vi "Test Section Cluster Tools.vi"() -> ()   [LabVIEW 2015]
uses:
  JSONtext.lvlib
panel:
  out "data":cluster{"3124":i32, "efqwf":string}
  out "error out":errorcluster
  out "<JSON>":string
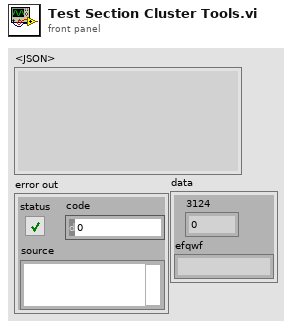
[diagram p1: front panel]
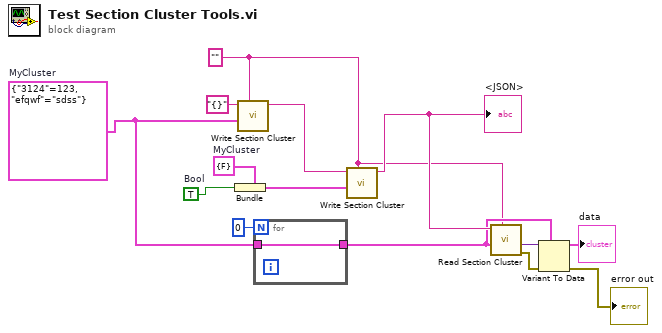
[diagram p0: block diagram]
diagram:
  w3 = cluster{"Bool":bool} {"Bool"=FALSE}  # MyCluster
  w1 = "" ("Path into Object")
  w12 = TRUE  # Bool
  w8 = cluster{"3124":i32, "efqwf":string} {"3124"=123, "efqwf"="sdss"}  # MyCluster
  n1 = Bundle(cluster=w3, "Bool"=w12) -> (w11:cluster{"Bool":bool})
  n2 = call "Write Section Cluster.vi"("Section Name (Cluster Name)"=w1, "Section Cluster"=w8, "JSON Object to merge into"="{}") -> ("<JSON>"=w13:string)  [unwired: 6 in, 1 out]
  n3 = for {
    N: 0 -> [_]
    tunnel: [w15] -> w4
    tunnel: w8 -> [w15]
  }
  n4 = call "Write Section Cluster.vi"("Section Name (Cluster Name)"=w1, "Section Cluster"=w11, "JSON Object to merge into"=w13) -> ("<JSON>"=w10:string)  [unwired: 6 in, 1 out]
  "<JSON>" <- w10
  n5 = call "Read Section Cluster.vi"("Section (Cluster Name)"=w1, "Cluster"=w4, "JSON Object"=w10) -> ("error out"=w6:errorcluster, "Cluster set from section"=w7:variant)  [unwired: 5 in, 1 out]
  n6 = Variant To Data(error in=w6, type=w4, Variant=w7) -> (data=→"data":cluster{"3124":i32, "efqwf":string}, error out=→"error out":errorcluster)
